vi "Dialog.vi"(0 "Message":string, 1 "Title":string, 5 "LeftButtonText(\"Yes\")":string="Yes", 7 "MiddleButtonText(\"No\")":string="No", 9 "RightButtonText(\"Cancel\")":string="Cancel", 11 "error in":errorcluster, 12 "CheckboxText":string="Remember my choice (can be changed by deleting the lvdelete.ini file)") -> (4 "Enum":T1, 8 "Checked?":bool, 15 "error out":errorcluster)   [LabVIEW 2020]
doc: "Created by Bas v. Etten 2024"
uses:
  ButtonDialogEnum.ctl
panel:
  in  "Checkbox":bool
  in  "Right Button":bool
  in  "MiddleButton":bool
  in  "LeftButton":bool
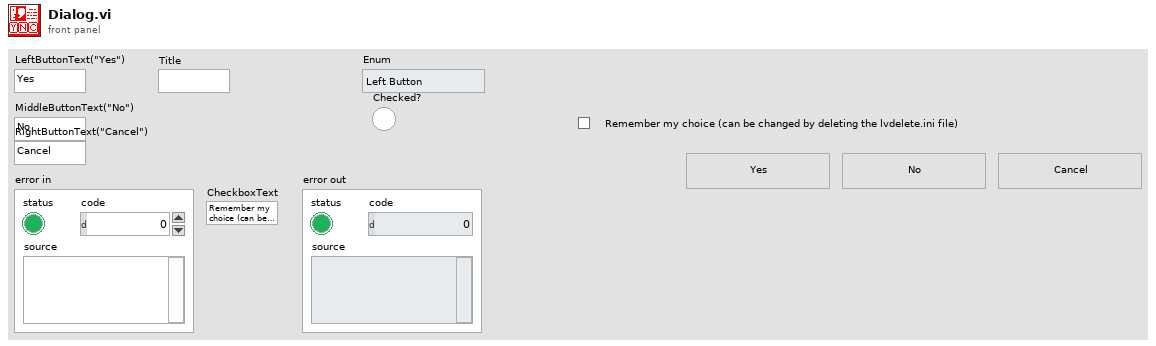
[diagram p1: front panel]
types:
  T1 = typedef "ButtonDialogEnum.ctl" = enum16{"Left Button", "Middle Button", "Right Button", "Window Close"}
  T2 = enum16{"Left Button", "Middle Button", "Right Button", "Window Close"}
  T3 = enum16{"Left Button", "Middle Button", "Right Button"}
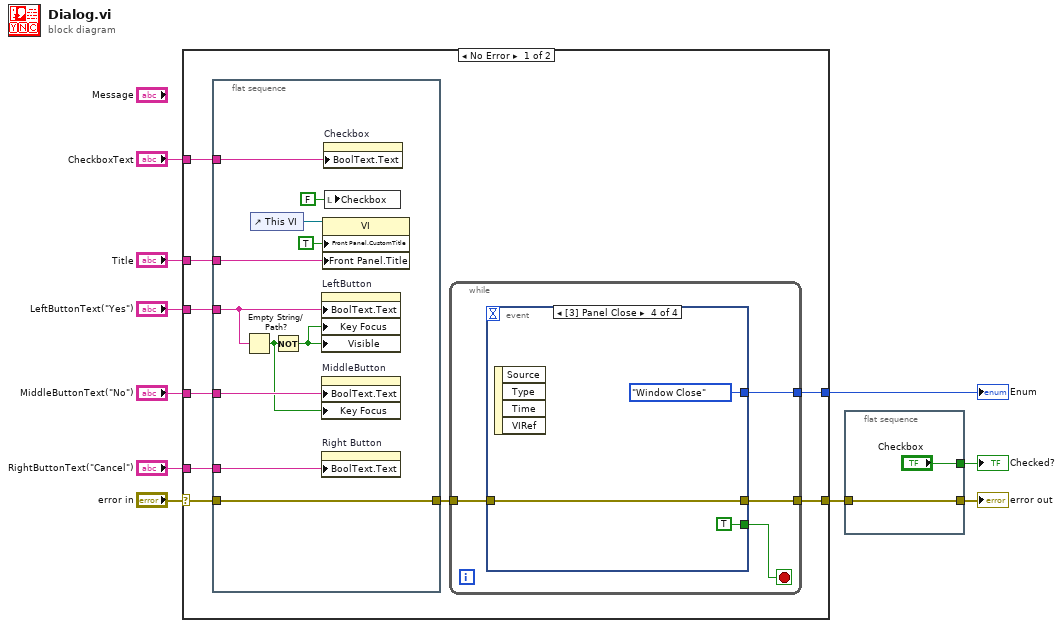
[diagram p0: block diagram]
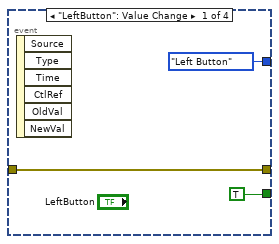
[diagram p2: hidden frame]
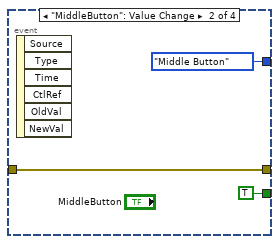
[diagram p3: hidden frame]
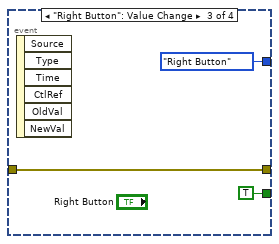
[diagram p4: hidden frame]
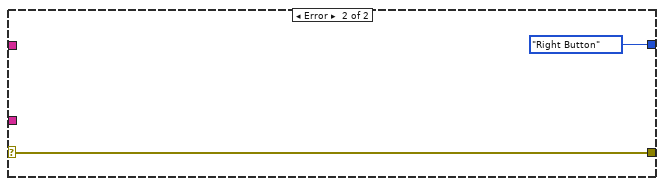
[diagram p5: hidden frame]
diagram:
  n1 = case shown="No Error" "error in" {
    selector: "error in" -> [w18 w48]
    tunnel: [w19 w48] -> w3
    tunnel: [w16 T3."Right Button" ("Enum")] -> w9
    tunnel: "Title" -> [w12 _]
    tunnel: "RightButtonText(\"Cancel\")" -> [w15 _]
    tunnel: "MiddleButtonText(\"No\")" -> [w14 _]
    tunnel: "LeftButtonText(\"Yes\")" -> [w13 _]
    tunnel: "CheckboxText" -> [w11 _]
    frame No Error {
      n2 = flat-sequence {
        tunnel: w18 -> [w30]
        tunnel: [w30] -> w17
        tunnel: w15 -> [w29]
        tunnel: w14 -> [w28]
        tunnel: w13 -> [w22]
        tunnel: w12 -> [w25]
        tunnel: w11 -> [w23]
        frame #0 {
          n3 = Empty String/Path?(string/path=w22) -> (empty?=w20:bool)
          n4 = control-ref of="This VI"() -> (w27:refnum<vi>)
          n5 = Not(x=w20) -> (.not. x?=w21:bool)
          n6 = property on="LeftButton" class="Bool"("BoolText.Text"=w22, "Key Focus"=w21, "Visible"=w21) -> ()  [unwired: 2 in, 2 out]
          n7 = property on="MiddleButton" class="Bool"("BoolText.Text"=w28, "Key Focus"=w20) -> ()  [unwired: 2 in, 2 out]
          n8 = property on="Right Button" class="Bool"("BoolText.Text"=w29) -> ()  [unwired: 2 in, 2 out]
          n9 = property class="VI"(reference=w27, "Front Panel.CustomTitle"=TRUE ("Front Panel Window:Custom Title"), "Front Panel.Title"=w25) -> ()  [unwired: 1 in, 2 out]
          n10 = property on="Checkbox" class="Bool (strict)"("BoolText.Text"=w23) -> ()  [unwired: 2 in, 2 out]
          n11 = local write "Checkbox"(FALSE ("Checkbox")) -> ()
        }
      }
      n12 = while {
        tunnel: [w33] -> w19
        tunnel: w17 -> [w32]
        tunnel: [w31] -> w16
        stop <- w34 stop-if-true
        n13 = event shown="[3] Panel Close" {
          selector: _ -> [_ _ _ _]
          dyn-events: _ -> [_ _ _ _]
          timeout: _ -> [_ _ _ _]
          tunnel: [TRUE TRUE TRUE TRUE] -> w34
          tunnel: [w36 w40 w43 w46] -> w33
          tunnel: w32 -> [w36 w40 w43 w46]
          tunnel: [T2."Left Button" ("Enum") T2."Middle Button" ("Enum") T2."Right Button" ("Enum") T2."Window Close" ("Enum")] -> w31
          event "LeftButton": Value Change {
            n14 = event-data() -> ()  [unwired: 1 in, 6 out]
          }
          event "MiddleButton": Value Change {
            n15 = event-data() -> ()  [unwired: 1 in, 6 out]
          }
          event "Right Button": Value Change {
            n16 = event-data() -> ()  [unwired: 1 in, 6 out]
          }
          event Panel Close {
            n17 = event-data() -> ()  [unwired: 1 in, 4 out]
          }
        }
      }
    }
    frame Error {
    }
  }
  "Enum" <- w9
  n18 = flat-sequence {
    tunnel: w3 -> [w50]
    tunnel: [w50] -> w2
    tunnel: ["Checkbox"] -> w1
    frame #0 {
    }
  }
  "error out" <- w2
  "Checked?" <- w1
